vi "LSX Get Snapshot Pos.vi"(0 "lLSID":i32, 1 "pdA":dbl, 5 "pdX":dbl, 7 "pdY":dbl, 9 "pdZ":dbl, 11 "error in (no error)":errorcluster) -> (3 "pdA out":dbl, 4 "function return":i32, 6 "pdX out":dbl, 8 "pdY out":dbl, 10 "pdZ out":dbl, 15 "error out":errorcluster)   [LabVIEW 2016, in "Tango_DLL.lvlib"]
doc: "TANGOAPI int TANGOCALL LSX_GetSnapshotPos (int lLSID, double *pdX, double *pdY, double *pdZ, double *pdA);"
uses:
  Tango_DLL.lvlib
  2017/Microscope Control/Device Library/Stages/Marzhauser/SCAN IM 120 x 80/Tango DLL VIs/Tango_DLL.dll
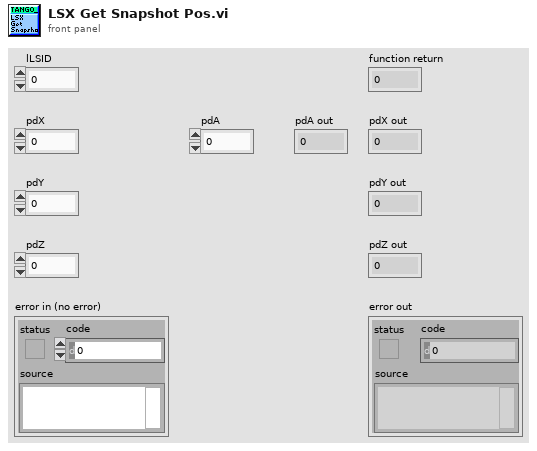
[diagram p1: front panel]
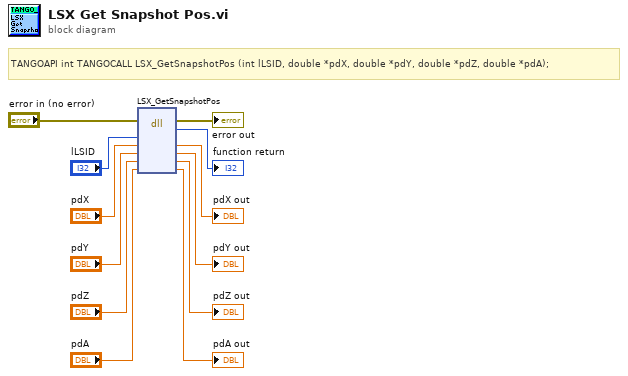
[diagram p0: block diagram]
diagram:
  # "TANGOAPI int TANGOCALL LSX_GetSnapshotPos (int lLSID, double *pdX, double *pdY, double *pdZ, double *pdA);"
  n1 = dll-call lib="C:/Users/4PiSMS/Documents/Microscope Control/2017/Microscope Control/Device Library/Stages/Marzhauser/SCAN IM 120 x 80/Tango DLL VIs/Tango_DLL.*" fn="LSX_GetSnapshotPos"(error in="error in (no error)", "lLSID"="lLSID", "pdX"="pdX", "pdY"="pdY", "pdZ"="pdZ", "pdA"="pdA") -> (error out=→"error out":errorcluster, →"function return":i32, "pdX"=→"pdX out":dbl, "pdY"=→"pdY out":dbl, "pdZ"=→"pdZ out":dbl, "pdA"=→"pdA out":dbl)  [unwired: 3 in, 1 out]
